vi "Get Data content.vi"(4 "error in (no error)":errorcluster, 6 "Data in":refnum<class "Data.lvclass">) -> (0 "error out":errorcluster, 2 "Data out":refnum<class "Data.lvclass">, 3 "Data Content":sgl[][](array[numeric]))   [LabVIEW 2018]
doc: "Displays the content of a Data object containing 2-dimensional OCT data, in an intensity graph. The refractive index can be specified to account for skew in the z axis.\nThe raw image data is returned in a 2D array of single."
uses:
  SpectralRadar/LabVIEW/2012/user.lib/SpectralRadar.llb/Data.lvclass
  SpectralRadar/LabVIEW/2012/user.lib/SpectralRadar.llb/Data Property Int Selection.ctl
  SpectralRadar/LabVIEW/2012/user.lib/SpectralRadar.llb/get Data Property Int.vi
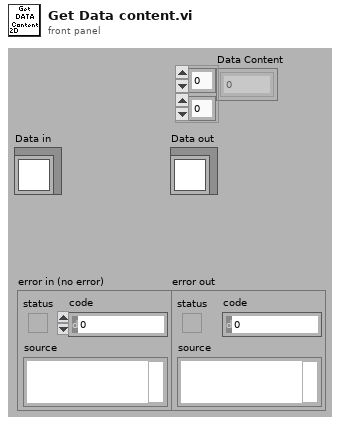
[diagram p1: front panel]
types:
  T1 = typedef "Data.lvclass/Data Property Int Selection.ctl" = enum16{"Dimensions", "Size 1", "Size 2", "Size 3", "Number of Data Points", "Data Size in Bytes", "Bytes per Pixel"}
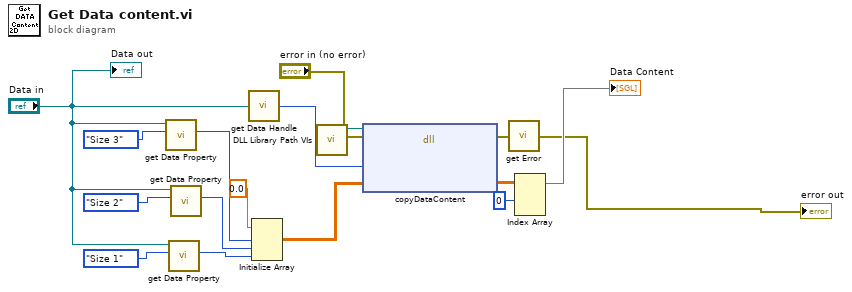
[diagram p0: block diagram]
diagram:
  n1 = call-poly "get Data Property.vi"("Data Property Selection"=Data_Property_Int_Selection."Size 3", "Data"="Data in") -> ("Property Value"=w4:i32)  [unwired: 3 in, 2 out]
  n2 = call-poly "get Data Property.vi"("Data Property Selection"=Data_Property_Int_Selection."Size 1", "Data"="Data in") -> ("Property Value"=w10:i32)  [unwired: 3 in, 2 out]
  n3 = call-poly "get Data Property.vi"("Data Property Selection"=Data_Property_Int_Selection."Size 2", "Data"="Data in") -> ("Property Value"=w9:i32)  [unwired: 3 in, 2 out]
  n4 = call "get Data Handle.vi"("Data"="Data in") -> ("Handle"=w16:u64)
  n5 = Initialize Array(sgl 0.0 ("element"), w4, w9, w10) -> (w15:sgl[][][])
  n6 = call "DLL Library Path VIs.vi"() -> ("SpectralRadarDLL"=w1:path)  [unwired: 8 in, 3 out]
  n7 = dll-call lib="C:/Project/SerialSectOCT - FFT GPU/SerialSectOCT/Labview Software/DLL/SpectralRadar.dll" fn="copyDataContent"(path in=w1, error in="error in (no error)", "Data Handle"=w16, "Data Content"=w15) -> (error out=w8:errorcluster, "Data Content"=w14:sgl[][][])  [unwired: 3 in, 1 out]
  n8 = call "get Error.vi"("error in (no error)"=w8) -> ("error out"=→"error out":errorcluster)
  n9 = Index Array(array=w14, index (dim 0)=0 ("index (page)")) -> (element=→"Data Content":sgl[][])  [unwired: 2 in]
  "Data out" <- "Data in"
